vi "Split HDC Bank2 DIO.vi"(7 "IN 7:0":u8 format="%08b") -> (0 "OUT 5":bool, 1 "OUT 7:6":fxp<+,2,2> format="%02b", 2 "OUT 4:3":fxp<+,2,2> format="%02b", 3 "OUT 2":bool, 4 "OUT 0":bool, 5 "OUT 1":bool)   [LabVIEW 2017]
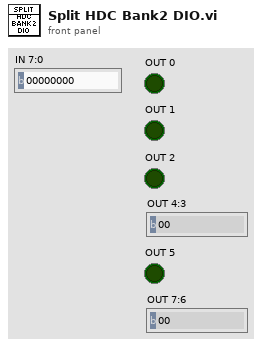
[diagram p1: front panel]
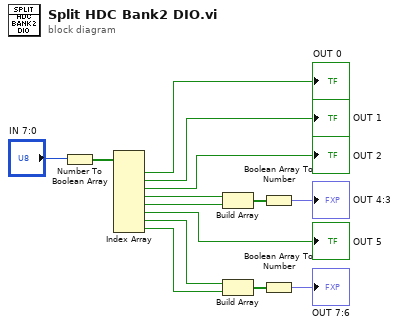
[diagram p0: block diagram]
diagram:
  n1 = Number To Boolean Array(number="IN 7:0") -> (Boolean array=w13:bool[])
  n2 = Index Array(array=w13) -> (element #1=→"OUT 0":bool, element #2=→"OUT 1":bool, element #3=→"OUT 2":bool, element #4=w3:bool, element #5=w2:bool, element #6=→"OUT 5":bool, element #7=w12:bool, element #8=w11:bool)  [unwired: 8 in]
  n3 = Build Array(w3, w2) -> (w4:bool[])
  n4 = Build Array(w12, w11) -> (w10:bool[])
  n5 = Boolean Array To Number(Boolean array=w4) -> (number=→"OUT 4:3":fxp<+,2,2>)
  n6 = Boolean Array To Number(Boolean array=w10) -> (number=→"OUT 7:6":fxp<+,2,2>)
